vi "From String.vi"(8 "error in (no error)":errorcluster, 9 "initial scan location":u32, 10 "String":string, 11 "Double Float in":refnum<class "Abs_Double Float.lvclass">) -> (0 "error out":errorcluster, 1 "offset past scan":u32, 2 "Remaining String":string, 3 "Double Float out":refnum<class "Abs_Double Float.lvclass">)   [LabVIEW 2021, in "Abs_Double Float.lvclass"]
uses:
  Abs_Double Float.lvclass
  C:/Program Files (x86)/National Instruments/LabVIEW 2021/vi.lib/TSA/Abstract Data Classes/Abs_Types/Numeric/Abs_Numeric.lvclass
  Support/Type.ctl
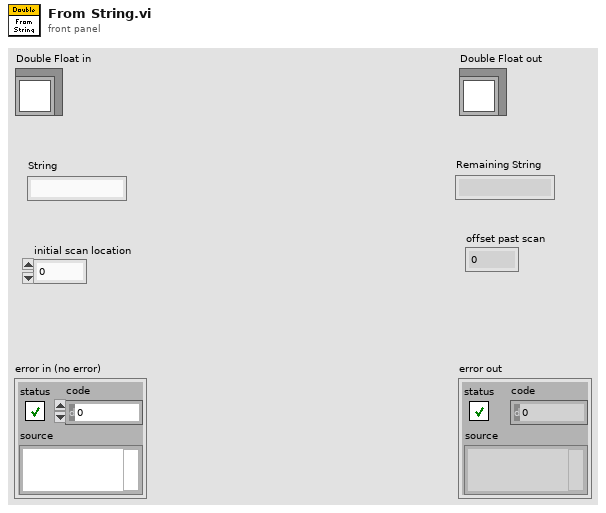
[diagram p1: front panel]
types:
  T1 = typedef "Abs_Double Float.lvclass/Type.ctl" = dbl
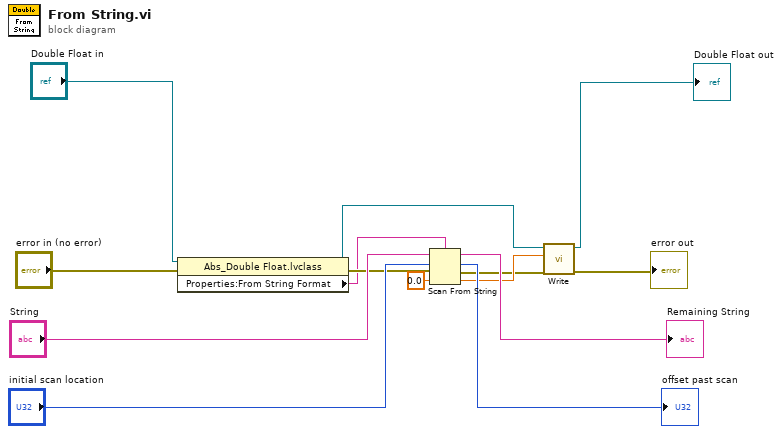
[diagram p0: block diagram]
diagram:
  n1 = property class="Abs_Double Float.lvclass"(reference="Double Float in", error in="error in (no error)") -> (reference out=w1:refnum<class "Abs_Double Float.lvclass">, error out=w4:errorcluster, "Properties:From String Format"=w3:string)
  n2 = Scan From String(format string=w3, input string="String", initial scan location="initial scan location", error in=w4, default 1=T1 0.0 ("default value 1")) -> (remaining string=→"Remaining String":string, offset past scan=→"offset past scan":u32, error out=w5:errorcluster, output 1=w6:T1)
  n3 = call-dynamic "Write.vi"("error in (no error)"=w5, "Value"=w6, "Double Float.lvclass in"=w1) -> ("error out"=→"error out":errorcluster, "Double Float.lvclass out"=→"Double Float out":refnum<class "Abs_Double Float.lvclass">)  [unwired: 7 in]
